vi "InitQueue.vi"   [LabVIEW 2013]
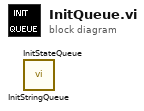
[diagram p0: block diagram]
diagram:
  n1 = call "InitStringQueue.vi"() -> ()  [unwired: 10 in, 2 out]
  n2 = call "InitStateQueue.vi"() -> ()  [unwired: 10 in, 2 out]
